vi "Configure Math.vi"(0 "VISA resource name":refnum<visa-resource-name>, 1 "Calculation 1 (0: Off)":u16(ring) items=["Off", "MX+B", "Percent"], 2 "Calculation 2 (0: Off)":u16(ring) items=["Off", "Minimum", "Maximum", "Mean", "Standard Deviation"], 3 "Calculation 3 (0: Off)":u16(ring) items=["Off", "Limit"], 5 "error in (no error)":errorcluster, 6 "Slope (M) (1.00000)":dbl=1.0 format="%_6g", 7 "Lower Limit (-1.00000)":dbl=-1.0 format="%_6g", 8 "Offset (B) (0.00000)":dbl format="%_6g", 9 "Upper Limit (1.00000)":dbl=1.0 format="%_6g", 10 "Percent Reference (1.00000)":dbl=1.0 format="%_6g") -> (14 "VISA resource name out":refnum<visa-resource-name>, 19 "error out":errorcluster)   [LabVIEW 2009, in "Keithley 2000.lvlib"]
doc: "This VI configures the math functions of the instrument. This includes MX+B, Percent, Minimum, Maximum, Mean, Standard Deviation, and Limits calculations."
uses:
  <instrlib>/Keithley 2000/Keithley 2000.lvlib
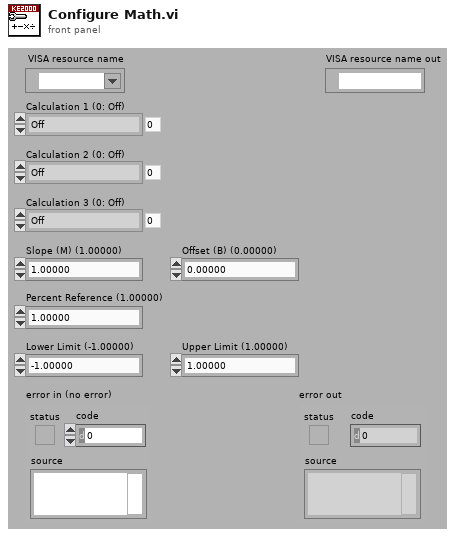
[diagram p1: front panel]
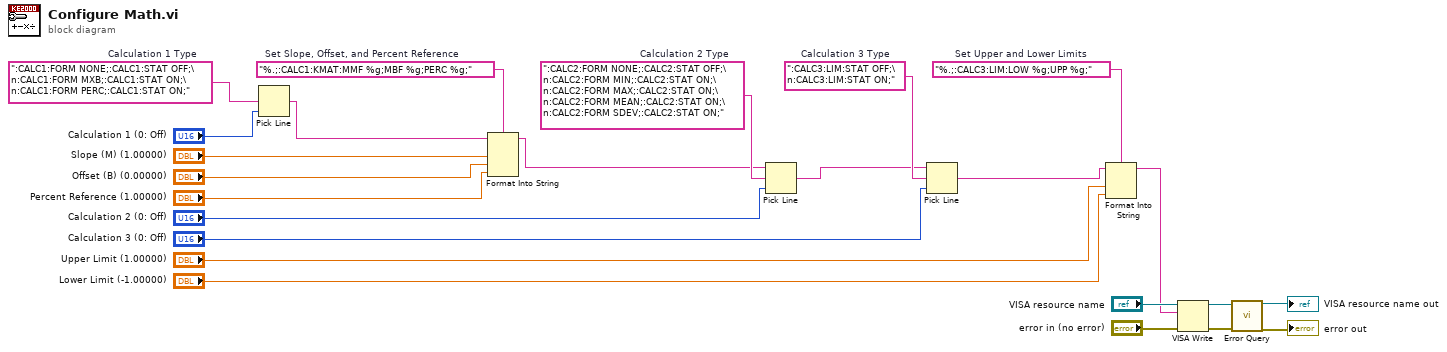
[diagram p0: block diagram]
diagram:
  w9 = "%.;:CALC3:LIM:LOW %g;UPP %g;"  # Set Upper and Lower Limits
  w12 = ":CALC3:LIM:STAT OFF;\n:CALC3:LIM:STAT ON;"  # Calculation 3 Type
  w15 = ":CALC2:FORM NONE;:CALC2:STAT OFF;\n:CALC2:FORM MIN;:CALC2:STAT ON;\n:CALC2:FORM MAX;:CALC2:STAT ON;\n:CALC2:FORM MEAN;:CALC2:STAT ON;\n:CALC2:FORM SDEV;:CALC2:STAT ON;"  # Calculation 2 Type
  w20 = "%.;:CALC1:KMAT:MMF %g;MBF %g;PERC %g;"  # Set Slope, Offset, and Percent Reference
  w22 = ":CALC1:FORM NONE;:CALC1:STAT OFF;\n:CALC1:FORM MXB;:CALC1:STAT ON;\n:CALC1:FORM PERC;:CALC1:STAT ON;"  # Calculation 1 Type
  n1 = Pick Line(multi-line string=w22, line index="Calculation 1 (0: Off)") -> (output string=w19:string)  [unwired: 1 in]
  n2 = Format Into String(format string=w20, initial string=w19, "Slope (M) (1.00000)", "Offset (B) (0.00000)", "Percent Reference (1.00000)") -> (resulting string=w14:string)  [unwired: 1 in, 1 out]
  n3 = Pick Line(string ("")=w14, multi-line string=w15, line index="Calculation 2 (0: Off)") -> (output string=w11:string)
  n4 = Pick Line(string ("")=w11, multi-line string=w12, line index="Calculation 3 (0: Off)") -> (output string=w8:string)
  n5 = Format Into String(format string=w9, initial string=w8, "Upper Limit (1.00000)", "Lower Limit (-1.00000)") -> (resulting string=w5:string)  [unwired: 1 in, 1 out]
  n6 = VISA Write(VISA resource name="VISA resource name", write buffer=w5, error in (no error)="error in (no error)") -> (VISA resource name out=w4:refnum<visa-resource-name>, error out=w1:errorcluster)  [unwired: 1 out]
  n7 = call <instrlib>:"Error Query.vi"("VISA resource name"=w4, "error in (no error)"=w1) -> ("VISA resource name out"=→"VISA resource name out":refnum<visa-resource-name>, "error out"=→"error out":errorcluster)  [unwired: 14 in, 2 out]
